vi "Handle Request.vi"(7 "Processing In":refnum<class "Processing.lvclass">, 11 "Authentication Handler in":refnum<class "Authentication Handler.lvclass">) -> (0 "error out":errorcluster, 5 "Processing":refnum<class "Processing.lvclass">)   [LabVIEW 2020, in "HTTP Server.lvlib" / "Authentication Handler.lvclass"]
uses:
  Authentication Handler.lvclass
  Processing/Processing.lvclass
  User Provider/User Provider.lvclass
  C:/dev/lv20CE/relink/lv-http-server/HTTP Server/Service/Service.lvclass
  Security/Security.lvclass
  Authentication Provider/Authentication Provider.lvclass
  Processing/Processing.lvclass/Processing.ctl
  lv-http-util/HTTP Utils/Response/Response.lvclass
  Password Encoder/Password Encoder.lvclass
  Authentication Inputs.ctl
  lv-http-util/HTTP Utils/Request/Request.lvclass
  Session/Session.lvclass
  lv-http-util/HTTP Utils/Redirect Response/Redirect Response.lvclass
  C:/dev/lv20CE/relink/lv-http-util/HTTP Utils/Response/Response.lvclass
  lv-http-util/HTTP Utils/Request/Get Target URI.vi
  lv-stream/stream/URI/Get Path.vi
  Authentication Handler.lvclass/Authentication Handler.ctl
  HTTP Server.lvlib
  User/User.lvclass
  C:/dev/lv20CE/relink/lv-http-server/HTTP Server/Security/Security.lvclass
  Values/Values.lvclass
  lv-uri/URI/URI/URI.lvclass
  C:/dev/lv20CE/relink/lv-http-util/HTTP Utils/Redirect Response/Redirect Response.lvclass
  C:/dev/lv20CE/relink/lv-http-server/HTTP Server/Password Encoder/Password Encoder.lvclass
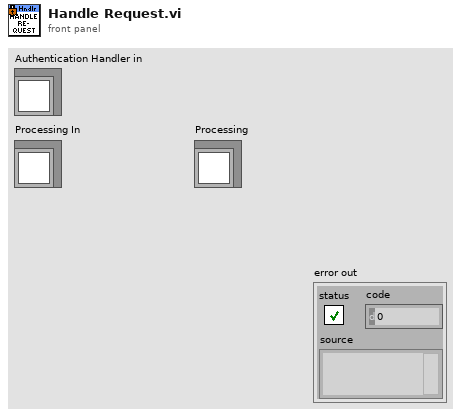
[diagram p1: front panel]
types:
  T1 = typedef "HTTP Server.lvlib/Authentication Inputs.ctl" = cluster{"Request":refnum<class "Request.lvclass">, "Session":refnum<class "Session.lvclass">, "User Provider":refnum<class "User Provider.lvclass">, "Password Encoder":refnum<class "Password Encoder.lvclass">}
  T2 = typedef "HTTP Server.lvlib/Authentication Outputs.ctl" = cluster{"User":refnum<class "User.lvclass">, "Session":refnum<class "Session.lvclass">}
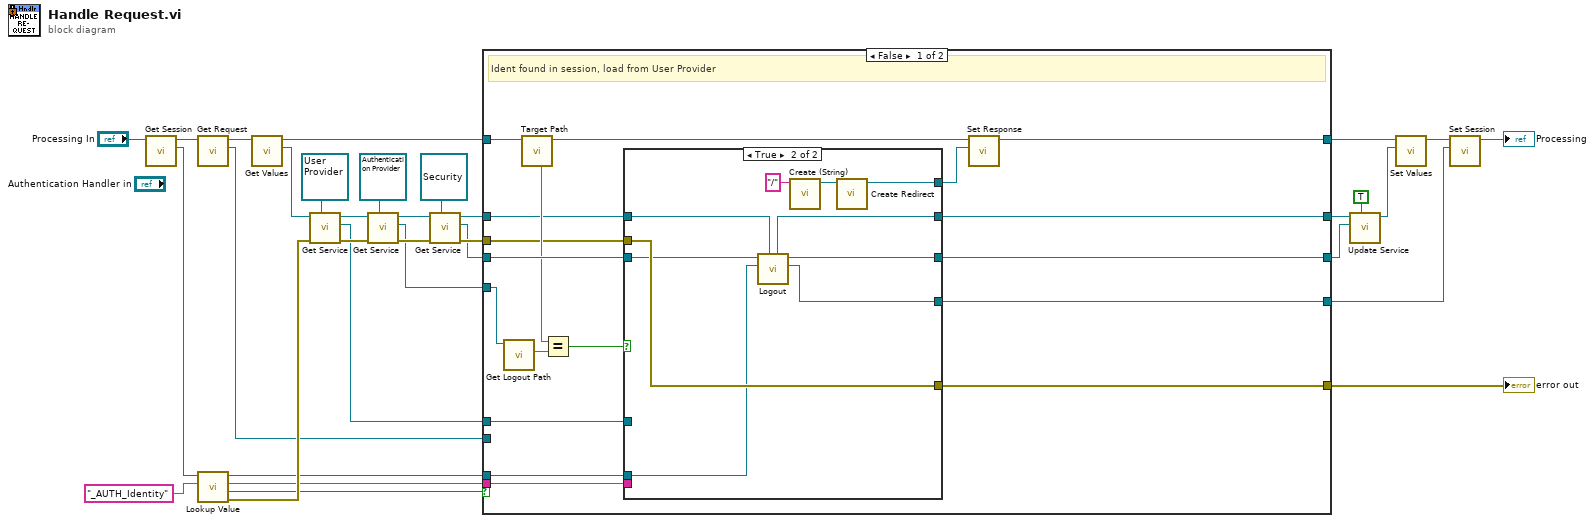
[diagram p0: block diagram]
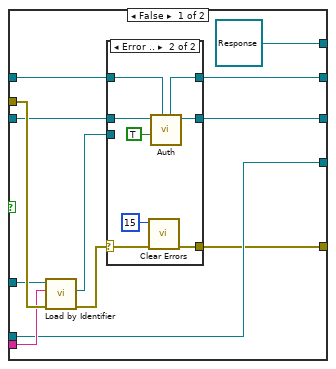
[diagram p2: hidden frame]
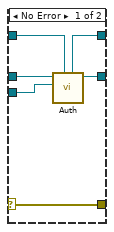
[diagram p3: hidden frame]
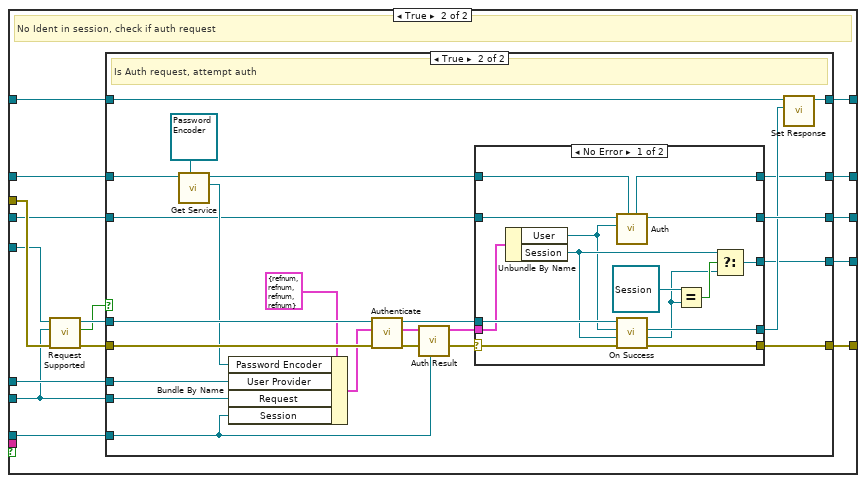
[diagram p4: hidden frame]
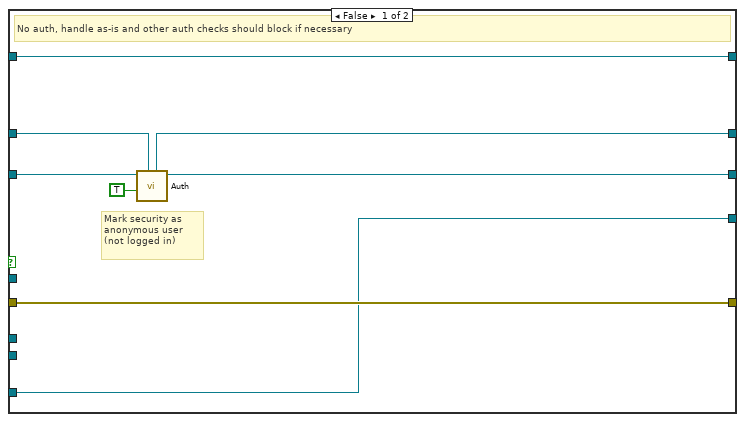
[diagram p5: hidden frame]
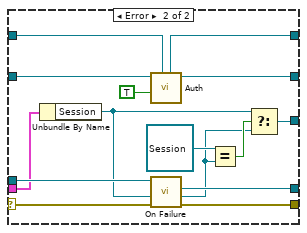
[diagram p6: hidden frame]
diagram:
  n1 = call "Get Session.vi"("Processing in"="Processing In") -> ("Session"=w12:refnum<class "Session.lvclass">, "Processing out"=w2:refnum<class "Processing.lvclass">)  [unwired: 9 in]
  n2 = call "Get Request.vi"("Processing in"=w2) -> ("Request"=w3:refnum<class "Request.lvclass">, "Processing out"=w1:refnum<class "Processing.lvclass">)  [unwired: 9 in]
  n3 = call "Lookup Value.vi"("Name"="_AUTH_Identity", "Session in"=w12) -> ("error out"=w30:errorcluster, "Not Found?"=w29:bool, "Value"=w28:string, "Session out"=w26:refnum<class "Session.lvclass">)  [unwired: 6 in]
  n4 = call "Get Values.vi"("Processing in"=w1) -> ("Values"=w11:refnum<class "Values.lvclass">, "Processing out"=w8:refnum<class "Processing.lvclass">)  [unwired: 9 in]
  n5 = call "Get Service.vi"("Service Type"=refnum<class "User Provider.lvclass"> refnum ("HTTP Server.lvlib:User Provider.lvclass"), "error in (no error)"=w30, "Values in"=w11) -> ("error out"=w33:errorcluster, "Service"=w27:refnum<class "User Provider.lvclass">, "Values out"=w17:refnum<class "Values.lvclass">)  [unwired: 6 in]
  n6 = call "Get Service.vi"("Service Type"=refnum<class "Authentication Provider.lvclass"> refnum ("HTTP Server.lvlib:Authentication Provider.lvclass"), "error in (no error)"=w33, "Values in"=w17) -> ("error out"=w15:errorcluster, "Service"=w14:refnum<class "Authentication Provider.lvclass">, "Values out"=w16:refnum<class "Values.lvclass">)  [unwired: 6 in]
  n7 = call "Get Service.vi"("Service Type"=refnum<class "Security.lvclass"> refnum ("HTTP Server.lvlib:Security.lvclass"), "error in (no error)"=w15, "Values in"=w16) -> ("error out"=w32:errorcluster, "Service"=w23:refnum<class "Security.lvclass">, "Values out"=w22:refnum<class "Values.lvclass">)  [unwired: 6 in]
  n8 = case shown="False" w29 {
    tunnel: w28 -> [w51 _]
    tunnel: w27 -> [w48 w98]
    tunnel: w22 -> [w37 w92]
    tunnel: w32 -> [w36 w103]
    tunnel: [w34 w100] -> w10
    tunnel: w26 -> [w44 w99]
    tunnel: w23 -> [w50 w96]
    tunnel: [w49 w95] -> w20
    tunnel: [w35 w94] -> w19
    tunnel: w14 -> [w47 w93]
    tunnel: w8 -> [w40 w91]
    tunnel: [w42 w90] -> w7
    tunnel: [w41 w89] -> w4
    tunnel: w3 -> [_ w88]
    frame False {
      # "Ident found in session, load from User Provider"
      n9 = call-dynamic "Get Logout Path.vi"("Authentication Provider in"=w47) -> ("Logout Path"=w46:string)  [unwired: 8 in, 2 out]
      n10 = call "Target Path.vi"("Processing in"=w40) -> ("Processing out"=w38:refnum<class "Processing.lvclass">, "Target Path"=w39:string)  [unwired: 9 in]
      n11 = Equal?(x=w39, y=w46) -> (x = y?=w45:bool)
      n12 = case shown="True" w45 {
        tunnel: w51 -> [w62 _]
        tunnel: w50 -> [w60 w86]
        tunnel: [w59 w82] -> w49
        tunnel: w48 -> [w58 _]
        tunnel: w44 -> [w56 w85]
        tunnel: [w56 w84] -> w41
        tunnel: [refnum<class "Response.lvclass"> refnum ("Early Response") w80] -> w43
        tunnel: w37 -> [w55 w79]
        tunnel: [w54 w78] -> w35
        tunnel: w36 -> [w63 w87]
        tunnel: [w53 w87] -> w34
        frame False {
          n13 = call-dynamic "Load by Identifier.vi"("error in (no error)"=w63, "Identifier"=w62, "User Provider in"=w58) -> ("error out"=w61:errorcluster, "User"=w52:refnum<class "User.lvclass">)  [unwired: 6 in, 1 out]
          n14 = case shown="Error .." w61 {
            selector: w61 -> [w64 w77]
            tunnel: w52 -> [w67 _]
            tunnel: w60 -> [w69 w75]
            tunnel: [w68 w74] -> w59
            tunnel: w55 -> [w66 w71]
            tunnel: [w65 w70] -> w54
            tunnel: [w64 w72] -> w53
            frame No Error {
              n15 = call "Auth.vi"("Values In"=w66, "User (None)"=w67, "Security in"=w69) -> ("Security out"=w68:refnum<class "Security.lvclass">, "Values"=w65:refnum<class "Values.lvclass">)  [unwired: 6 in, 1 out]
            }
            frame Error {
              n16 = call <vilib>:"Clear Errors.vi"("error in (no error)"=w77, "specific error code to clear (0: all)"=15) -> ("error out"=w72:errorcluster)  [unwired: 4 in, 1 out]
              n17 = call "Auth.vi"("Values In"=w71, "Anonymous (F)"=TRUE, "Security in"=w75) -> ("Security out"=w74:refnum<class "Security.lvclass">, "Values"=w70:refnum<class "Values.lvclass">)  [unwired: 6 in, 1 out]
            }
          }
        }
        frame True {
          n18 = call "Logout.vi"("Values In"=w79, "Session In"=w85, "Security in"=w86) -> ("Session"=w84:refnum<class "Session.lvclass">, "Security out"=w82:refnum<class "Security.lvclass">, "Values"=w78:refnum<class "Values.lvclass">)  [unwired: 5 in, 1 out]
          n19 = call "Create (String).vi"("URI String"="/") -> ("URI out"=w81:refnum<class "URI.lvclass">)  [unwired: 9 in, 1 out]
          n20 = call "Create Redirect.vi"("Redirect URI"=w81) -> ("Redirect Response out"=w80:refnum<class "Redirect Response.lvclass">)  [unwired: 9 in, 1 out]
        }
      }
      n21 = call "Set Response.vi"("Response"=w43, "Processing in"=w38) -> ("Processing out"=w42:refnum<class "Processing.lvclass">)  [unwired: 9 in]
    }
    frame True {
      # "No Ident in session, check if auth request"
      n22 = call-dynamic "Request Supported.vi"("error in (no error)"=w103, "Request"=w88, "Authentication Provider in"=w93) -> ("error out"=w102:errorcluster, "Supported"=w97:bool, "Authentication Provider out"=w101:refnum<class "Authentication Provider.lvclass">)  [unwired: 6 in]
      n23 = case shown="True" w97 {
        tunnel: w92 -> [w106 w133]
        tunnel: w102 -> [w111 w131]
        tunnel: w101 -> [_ w132]
        tunnel: [w111 w114] -> w100
        tunnel: w99 -> [w107 w123]
        tunnel: w98 -> [_ w128]
        tunnel: w96 -> [w109 w121]
        tunnel: [w108 w120] -> w95
        tunnel: [w104 w115] -> w94
        tunnel: w91 -> [w105 w112]
        tunnel: [w105 w118] -> w90
        tunnel: [w107 w117] -> w89
        tunnel: w88 -> [_ w113]
        frame False {
          # "Mark security as anonymous user (not logged in)"
          # "No auth, handle as-is and other auth checks should block if necessary"
          n24 = call "Auth.vi"("Values In"=w106, "Anonymous (F)"=TRUE, "Security in"=w109) -> ("Security out"=w108:refnum<class "Security.lvclass">, "Values"=w104:refnum<class "Values.lvclass">)  [unwired: 6 in, 1 out]
        }
        frame True {
          # "Is Auth request, attempt auth"
          n25 = call "Get Service.vi"("Service Type"=refnum<class "Password Encoder.lvclass"> refnum ("HTTP Server.lvlib:Password Encoder.lvclass"), "Values in"=w133) -> ("Service"=w127:refnum<class "Password Encoder.lvclass">, "Values out"=w116:refnum<class "Values.lvclass">)  [unwired: 7 in, 1 out]
          n26 = Bundle By Name(cluster=T1 {"Request"=refnum, "Session"=refnum, "User Provider"=refnum, "Password Encoder"=refnum} ("Authentication Inputs"), "Password Encoder"=w127, "User Provider"=w128, "Request"=w113, "Session"=w123) -> (w129:T1)
          n27 = call-dynamic "Authenticate.vi"("error in (no error)"=w131, "Authentication Inputs"=w129, "Authentication Provider in"=w132) -> ("error out"=w126:errorcluster, "Authentication Outputs"=w124:T2, "Authentication Provider out"=w125:refnum<class "Authentication Provider.lvclass">)  [unwired: 6 in]
          n28 = call "Auth Result.vi"("Session In"=w123, "Authentication Outputs"=w124) -> ("Authentication Result"=w122:T2)  [unwired: 9 in]
          n29 = case shown="No Error" w126 {
            selector: w126 -> [w148 w163]
            tunnel: w122 -> [w145 w160]
            tunnel: [w140 w155] -> w117
            tunnel: w125 -> [w149 w164]
            tunnel: [w147 w162] -> w119
            tunnel: [w146 w161] -> w114
            tunnel: w121 -> [w139 w154]
            tunnel: [w137 w152] -> w120
            tunnel: w116 -> [w136 w151]
            tunnel: [w135 w150] -> w115
            frame No Error {
              n30 = Unbundle By Name(w145) -> ("User"=w138:refnum<class "User.lvclass">, "Session"=w141:refnum<class "Session.lvclass">)
              n31 = call "Auth.vi"("Values In"=w136, "User (None)"=w138, "Security in"=w139) -> ("Security out"=w137:refnum<class "Security.lvclass">, "Values"=w135:refnum<class "Values.lvclass">)  [unwired: 6 in, 1 out]
              n32 = call-dynamic "On Success.vi"("error in (no error)"=w148, "Session In"=w141, "User"=w138, "Authentication Provider in"=w149) -> ("error out"=w146:errorcluster, "Session"=w142:refnum<class "Session.lvclass">, "Response"=w147:refnum<class "Response.lvclass">)  [unwired: 4 in, 1 out]
              n33 = Equal?(x=refnum<class "Session.lvclass"> refnum, y=w142) -> (x = y?=w143:bool)
              n34 = Select(t=w141, s=w143, f=w142) -> (s? t:f=w140:refnum<class "Session.lvclass">)
            }
            frame Error {
              n35 = Unbundle By Name(w160) -> ("Session"=w156:refnum<class "Session.lvclass">)
              n36 = call "Auth.vi"("Values In"=w151, "Anonymous (F)"=TRUE, "Security in"=w154) -> ("Security out"=w152:refnum<class "Security.lvclass">, "Values"=w150:refnum<class "Values.lvclass">)  [unwired: 6 in, 1 out]
              n37 = call-dynamic "On Failure.vi"("error in (no error)"=w163, "Session In"=w156, "Authentication Provider in"=w164) -> ("error out"=w161:errorcluster, "Session"=w157:refnum<class "Session.lvclass">, "Response"=w162:refnum<class "Response.lvclass">)  [unwired: 5 in, 1 out]
              n38 = Equal?(x=refnum<class "Session.lvclass"> refnum, y=w157) -> (x = y?=w158:bool)
              n39 = Select(t=w156, s=w158, f=w157) -> (s? t:f=w155:refnum<class "Session.lvclass">)
            }
          }
          n40 = call "Set Response.vi"("Response"=w119, "Processing in"=w112) -> ("Processing out"=w118:refnum<class "Processing.lvclass">)  [unwired: 9 in]
        }
      }
    }
  }
  "error out" <- w10
  n41 = call "Update Service.vi"("Overwrite? (F)"=TRUE, "Service"=w20, "Values in"=w19) -> ("Values out"=w9:refnum<class "Values.lvclass">)  [unwired: 7 in, 1 out]
  n42 = call "Set Values.vi"("Values"=w9, "Processing in"=w7) -> ("Processing out"=w6:refnum<class "Processing.lvclass">)  [unwired: 9 in]
  n43 = call "Set Session.vi"("Session"=w4, "Processing in"=w6) -> ("Processing out"=→"Processing":refnum<class "Processing.lvclass">)  [unwired: 9 in]
